vi "DPID.vi"(8 "error in (no error)":errorcluster, 11 "Node Ptr":T2 format="%.0x") -> (0 "error out":errorcluster)   [LabVIEW 2015, in "Diagnostics Addon System Explorer.lvlib"]
uses:
  Diagnostics Addon System Explorer.lvlib
  <vilib>/NI Veristand/Custom Device API/Custom Device Item Ref.ctl
  Shared/DPID Periodic Rate.ctl
  <vilib>/NI Veristand/Custom Device Tools/Custom Device Utility Library/Search Direction.ctl
  Shared/FG Action.ctl
  Shared/GUID Lookup.vi
  <vilib>/NI Veristand/Custom Device API/NI VeriStand - Set Item Property.vi
  <vilib>/NI Veristand/Custom Device API/Set Item Property (U32).vi
  <vilib>/NI Veristand/Custom Device API/NI VeriStand - Get Item Property.vi
  <vilib>/NI Veristand/Custom Device API/Get Item Property (U32).vi
  <vilib>/NI Veristand/Custom Device API/Set Item Property (U32 Array).vi
  <vilib>/NI Veristand/Custom Device API/Get Item Property (U32 Array).vi
  <vilib>/NI Veristand/Custom Device Tools/Custom Device Utility Library/NI VeriStand - Search for Item by GUID.vi
  <vilib>/NI Veristand/Custom Device API/Custom Device API.lvlib
  <vilib>/NI Veristand/Custom Device Tools/Custom Device Utility Library/Custom Device Utility Library.lvlib
  Shared/Diagnostics Addon Shared.lvlib
panel:
  in  "Speed":T1
  in  "Description":string
  in  "ID":u8 format="%.0x"
  out "PIDs":i32(listbox)
  in  "SHDocVw.IWebBrowser":refnum<k7>(container)
  in  "Header":cluster{"Section Name":string}={"Section Name"="Custom Device Item Settings"}
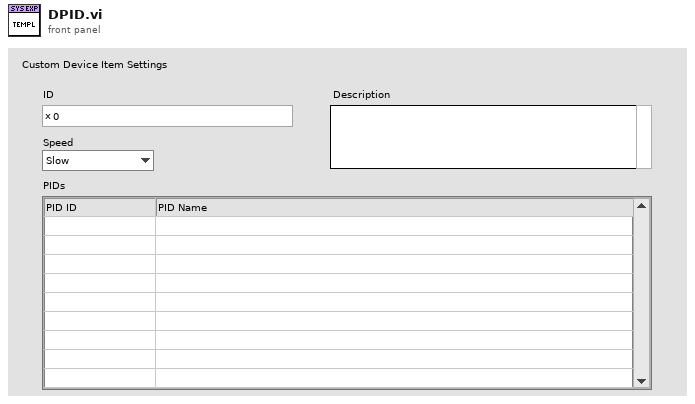
[diagram p1: front panel]
types:
  T1 = typedef "Diagnostics Addon Shared.lvlib/DPID Periodic Rate.ctl" = enum16{"Slow", "Medium", "Fast"}
  T2 = typedef "Custom Device API.lvlib/Custom Device Item Ref.ctl" = u64
  T3 = typedef "Diagnostics Addon System Explorer.lvlib/FG Action.ctl" = enum16{"Get", "Set"}
  T4 = typedef "Custom Device Utility Library.lvlib/Search Direction.ctl" = enum16{"Down", "Up"}
  T5 = typedef "Custom Device API.lvlib/Custom Device Item Info.ctl" = cluster{"Name":string, "Is Channel":bool, "GUID":string, "Is Waveform":bool}
  T6 = typedef "Diagnostics Addon Shared.lvlib/DPID Parameters.ctl" = cluster{"DPID ID":u8, "Speed":T1, "PIDs":u16[]}
  T7 = typedef "Custom Device API.lvlib/Custom Device Commands.ctl" = enum16{"Default", "Item renamed", "Shutdown", "Dynamic button pressed"}
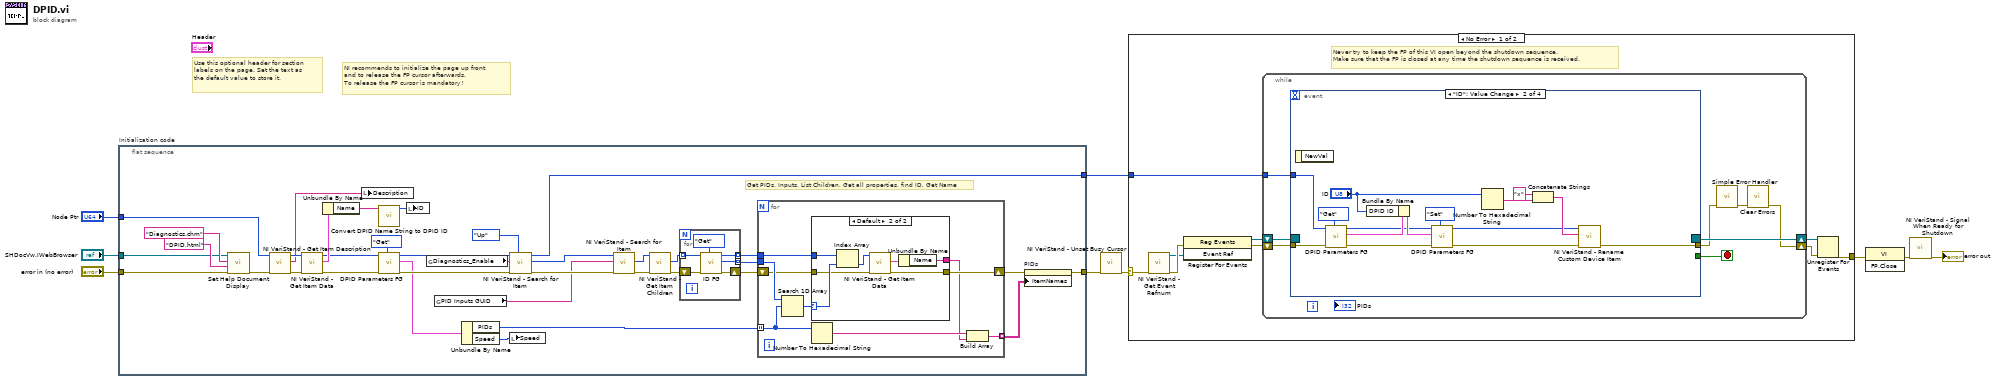
[diagram p0: block diagram]
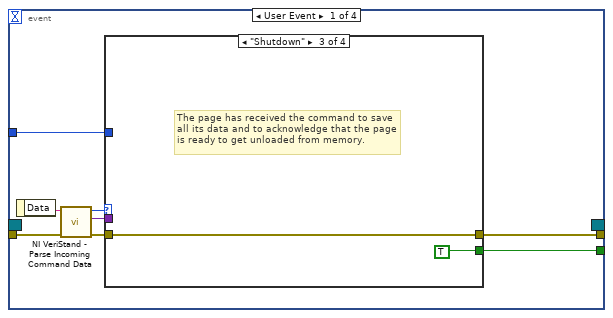
[diagram p2: hidden frame]
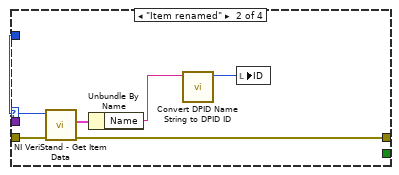
[diagram p4: hidden frame]
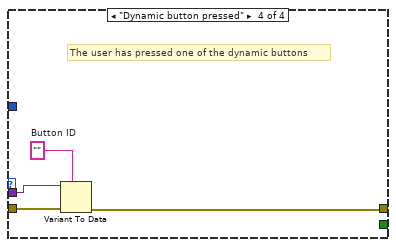
[diagram p5: hidden frame]
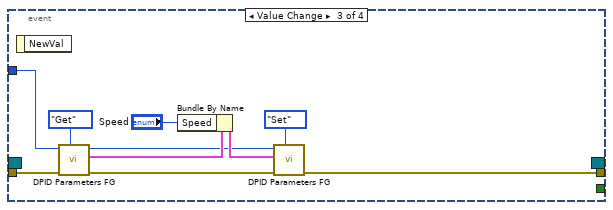
[diagram p6: hidden frame]
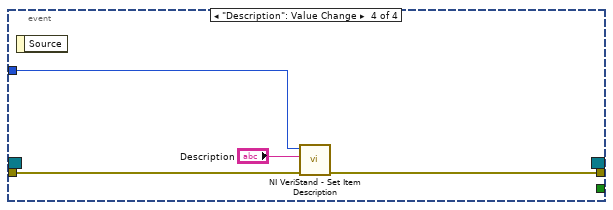
[diagram p7: hidden frame]
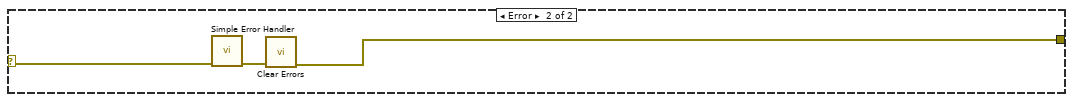
[diagram p8: hidden frame]
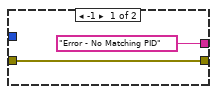
[diagram p9: hidden frame]
diagram:
  # "Use this optional header for section labels on the page. Set the text as the default value to store it."
  # "NI recommends to initialize the page up front\nand to release the FP cursor afterwards.\nTo release the FP cursor is mandatory!"
  n1 = flat-sequence "Initialization code" {
    tunnel: "error in (no error)" -> [w38]
    tunnel: "Node Ptr" -> [w44]
    tunnel: "SHDocVw.IWebBrowser" -> [w36]
    tunnel: [w30] -> w2
    tunnel: [w23] -> w1
    frame #0 {
      # "Get PIDs, Inputs, List Children, Get all properties, find ID, Get Name"
      n2 = call "Set Help Document Display.vi"("error in (no error)"=w38, "HTML File"="DPID.html", "Main CHM File"="Diagnostics.chm", "SHDocVw.IWebBrowser2"=w36) -> ("error out"=w37:errorcluster)  [unwired: 7 in]
      n3 = call <vilib>:"NI VeriStand - Get Item Description.vi"("error in (no error)"=w37, "Item Ref in"=w44) -> ("error out"=w42:errorcluster, "Description"=w43:string, "Item Ref out"=w45:T2)  [unwired: 7 out]
      n4 = call <vilib>:"NI VeriStand - Get Item Data.vi"("error in (no error)"=w42, "Item Ref in"=w45) -> ("error out"=w35:errorcluster, "Item Info"=w41:T5, "Item Ref out"=w34:T2)  [unwired: 7 out]
      n5 = Unbundle By Name(w41) -> ("Name"=w12:string)
      n6 = local write "Description"(w43) -> ()
      n7 = call "Convert DPID Name String to DPID ID.vi"("DPID Name"=w12) -> ("DPID ID"=w13:u8)  [unwired: 10 in]
      n8 = call "DPID Parameters FG.vi"("Action"=FG_Action."Get", "error in (no error)"=w35, "Device Item Ref in"=w34) -> ("error out"=w32:errorcluster, "DPID"=w29:T6, "Device Item Ref out"=w31:T2)  [unwired: 6 in]
      n9 = local write "ID"(w13) -> ()
      n10 = global read "GUID Lookup.vi" "Diagnostics_Enable"() -> (w33:string)
      n11 = global read "GUID Lookup.vi" "PID Inputs GUID"() -> (w18:string)
      n12 = Unbundle By Name(w29) -> ("PIDs"=w28:u16[], "Speed"=w11:T1)
      n13 = local write "Speed"(w11) -> ()
      n14 = call-poly <vilib>:"NI VeriStand - Search for Item.vi"("Direction (Down)"=Search_Direction."Up", "error in"=w32, "Item GUID"=w33, "Section Ref in"=w31) -> ("error out"=w19:errorcluster, "Item Ref"=w20:T2, "Section Ref out"=w30:T2)  [unwired: 4 in, 1 out]
      n15 = call-poly <vilib>:"NI VeriStand - Search for Item.vi"("error in"=w19, "Item GUID"=w18, "Section Ref in"=w20) -> ("error out"=w17:errorcluster, "Item Ref"=w15:T2)  [unwired: 5 in, 2 out]
      n16 = call <vilib>:"NI VeriStand - Get Item Children.vi"("error in (no error)"=w17, "Item Ref in"=w15) -> ("error out"=w16:errorcluster, "Child Refs"=w14:T2[])  [unwired: 6 in, 2 out]
      n17 = for {
        tunnel: w14 -> [w69] mode=indexing
        shift-right: [w67] -> w27
        shift-left: w16 -> [w68]
        tunnel: [w66] -> w25 mode=indexing
        tunnel: [w65] -> w26 mode=indexing
        n18 = call "ID FG.vi"("Action"=FG_Action."Get", "error in (no error)"=w68, "Device Item Ref in"=w69) -> ("error out"=w67:errorcluster, "ID"=w65:u32, "Device Item Ref out"=w66:T2)  [unwired: 6 in]
      }
      n19 = for {
        tunnel: w28 -> [w49] mode=indexing
        shift-right: [w50] -> w24
        shift-left: w27 -> [w51]
        tunnel: w26 -> [w54]
        tunnel: w25 -> [w53]
        tunnel: [w46] -> w22 mode=indexing
        n20 = Search 1D Array(1D array=w54, element=w49) -> (index of element=w52:i32)  [unwired: 1 in]
        n21 = case shown="Default" w52 {
          selector: w52 -> [_ w59]
          tunnel: ["Error - No Matching PID" ("Name") w62] -> w47
          tunnel: [w55 w61] -> w50
          tunnel: w53 -> [_ w60]
          tunnel: w51 -> [w55 w57]
          frame -1 {
          }
          frame Default {
            n22 = Index Array(array=w60, index=w59) -> (element=w58:T2)
            n23 = call <vilib>:"NI VeriStand - Get Item Data.vi"("error in (no error)"=w57, "Item Ref in"=w58) -> ("error out"=w61:errorcluster, "Item Info"=w63:T5)  [unwired: 8 out]
            n24 = Unbundle By Name(w63) -> ("Name"=w62:string)
          }
        }
        n25 = Number To Hexadecimal String(2:w49) -> (0:w48:string)  [unwired: 1 in]
        n26 = Build Array(w48, w47) -> (w46:string[])
      }
      n27 = property on="PIDs" class="MCListbox (strict)"(error in=w24, "ItemNames"=w22) -> (error out=w23:errorcluster)  [unwired: 1 in, 1 out]
    }
  }
  n28 = call <vilib>:"NI VeriStand - Unset Busy Cursor.vi"("error in (no error)"=w1) -> ("error out"=w5:errorcluster)  [unwired: 10 out]
  n29 = case shown="No Error" w5 {
    selector: w5 -> [w70 w139]
    tunnel: [w75 w137] -> w9
    tunnel: w2 -> [w71 _]
    frame No Error {
      # "Never try to keep the FP of this VI open beyond the shutdown sequence.\nMake sure that the FP is closed at any time the shutdown sequence is received."
      n30 = call <vilib>:"NI VeriStand - Get Event Refnum.vi"("error in (no error)"=w70) -> ("error out"=w78:errorcluster, "Event Ref"=w74:refnum<user-event>)  [unwired: 9 out]
      n31 = register-events(error in=w78, w74) -> (reference out=w72:refnum<event-registration>, error out=w73:errorcluster)  [unwired: 1 in]
      n32 = while {
        tunnel: w71 -> [w82]
        shift-right: [w79] -> w76
        shift-left: w73 -> [w85]
        shift-right: [w86] -> w77
        shift-left: w72 -> [w84]
        stop <- w83 stop-if-true
        n33 = event shown="[1] \"ID\": Value Change" {
          selector: w84 -> [_ _ _ _]
          dyn-events: [_ _ _ _] -> w86
          timeout: _ -> [_ _ _ _]
          tunnel: w85 -> [w94 w117 w132 w135]
          tunnel: [w90 _ _ _] -> w83
          tunnel: [w89 w122 w123 w134] -> w81
          tunnel: w82 -> [w88 w115 w131 w136]
          event User Event {
            n34 = event-data() -> ("Data"=w93:string)  [unwired: 1 out]
            n35 = call <vilib>:"NI VeriStand - Parse Incoming Command Data.vi"("error in (no error)"=w94, "Incoming data"=w93) -> ("error out"=w92:errorcluster, "Outgoing data"=w87:variant, "Action"=w91:T7)  [unwired: 7 out]
            n36 = case shown="\"Shutdown\"" w91 {
              tunnel: w92 -> [w95 w101 w102 w107]
              tunnel: [_ _ TRUE _] -> w90
              tunnel: [w95 w98 w102 w104] -> w89
              tunnel: w88 -> [_ w100 _ _]
              tunnel: w87 -> [_ _ _ w106]
              frame "Default", Default {
              }
              frame "Item renamed" {
                n37 = call <vilib>:"NI VeriStand - Get Item Data.vi"("error in (no error)"=w101, "Item Ref in"=w100) -> ("error out"=w98:errorcluster, "Item Info"=w99:T5)  [unwired: 8 out]
                n38 = Unbundle By Name(w99) -> ("Name"=w97:string)
                n39 = call "Convert DPID Name String to DPID ID.vi"("DPID Name"=w97) -> ("DPID ID"=w96:u8)  [unwired: 10 in]
                n40 = local write "ID"(w96) -> ()
              }
              frame "Shutdown" {
                # "The page has received the command to save all its data and to acknowledge that the page is ready to get unloaded from memory."
              }
              frame "Dynamic button pressed" {
                w105 = ""  # Button ID
                # "The user has pressed one of the dynamic buttons"
                n41 = Variant To Data(error in=w107, type=w105, Variant=w106) -> (error out=w104:errorcluster)  [unwired: 1 out]
              }
            }
          }
          event "ID": Value Change {
            n42 = event-data() -> ()  [unwired: 2 out]
            n43 = call "DPID Parameters FG.vi"("Action"=FG_Action."Get", "error in (no error)"=w117, "Device Item Ref in"=w115) -> ("error out"=w111:errorcluster, "DPID"=w118:T6, "Device Item Ref out"=w109:T2)  [unwired: 6 in]
            n44 = Bundle By Name(cluster=w118, "DPID ID"="ID") -> (w112:T6)
            n45 = call "DPID Parameters FG.vi"("Action"=FG_Action."Set", "error in (no error)"=w111, "DPID"=w112, "Device Item Ref in"=w109) -> ("error out"=w110:errorcluster, "Device Item Ref out"=w108:T2)  [unwired: 5 in, 1 out]
            n46 = Number To Hexadecimal String(2:"ID") -> (0:w121:string)  [unwired: 1 in]
            n47 = Concatenate Strings("x" ("element"), w121) -> (w119:string)
            n48 = call <vilib>:"NI VeriStand - Rename Custom Device Item.vi"("error in (no error)"=w110, "New Name"=w119, "Item Ref in"=w108) -> ("error out"=w122:errorcluster)  [unwired: 1 in, 7 out]
          }
          event Value Change {
            n49 = event-data() -> ()  [unwired: 2 out]
            n50 = call "DPID Parameters FG.vi"("Action"=FG_Action."Get", "error in (no error)"=w132, "Device Item Ref in"=w131) -> ("error out"=w124:errorcluster, "DPID"=w130:T6, "Device Item Ref out"=w125:T2)  [unwired: 6 in]
            n51 = Bundle By Name(cluster=w130, "Speed"="Speed") -> (w126:T6)
            n52 = call "DPID Parameters FG.vi"("Action"=FG_Action."Set", "error in (no error)"=w124, "DPID"=w126, "Device Item Ref in"=w125) -> ("error out"=w123:errorcluster)  [unwired: 5 in, 2 out]
          }
          event "Description": Value Change {
            n53 = event-data() -> ()  [unwired: 2 out]
            n54 = call <vilib>:"NI VeriStand - Set Item Description.vi"("error in (no error)"=w135, "Description"="Description", "Item Ref in"=w136) -> ("error out"=w134:errorcluster)  [unwired: 8 out]
          }
        }
        n55 = call <vilib>:"Simple Error Handler.vi"("error in (no error)"=w81) -> ("error out"=w80:errorcluster)  [unwired: 1 in, 7 out]
        n56 = call <vilib>:"Clear Errors.vi"("error in (no error)"=w80) -> ("error out"=w79:errorcluster)  [unwired: 1 in, 5 out]
      }
      n57 = Unregister For Events(event registration refnum=w77, error in=w76) -> (error out=w75:errorcluster)
    }
    frame Error {
      n58 = call <vilib>:"Simple Error Handler.vi"("error in (no error)"=w139) -> ("error out"=w138:errorcluster)  [unwired: 1 in, 7 out]
      n59 = call <vilib>:"Clear Errors.vi"("error in (no error)"=w138) -> ("error out"=w137:errorcluster)  [unwired: 1 in, 5 out]
    }
  }
  n60 = invoke class="VI" method="FP.Close"(error in=w9) -> (error out=w8:errorcluster)  [unwired: 2 in, 2 out]
  n61 = call <vilib>:"NI VeriStand - Signal When Ready for Shutdown.vi"("error in (no error)"=w8) -> ("error out"=→"error out":errorcluster)  [unwired: 10 out]
